vi "Receiver.vi"() -> ()   [LabVIEW 2019]
panel:
  in  "stop":bool
  out "Humdity":dbl
  out "Temperature":dbl
  # "Receiver"
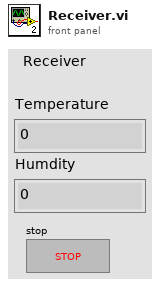
[diagram p1: front panel]
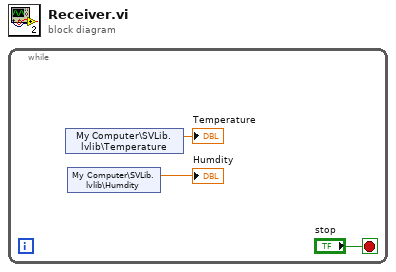
[diagram p0: block diagram]
diagram:
  n1 = while {
    stop <- "stop" stop-if-true
    n2 = shared-variable "My Computer\\SVLib.lvlib\\Temperature"() -> (→"Temperature":dbl)  [unwired: 1 in, 1 out]
    n3 = shared-variable "My Computer\\SVLib.lvlib\\Humdity"() -> (→"Humdity":dbl)  [unwired: 1 in, 1 out]
  }
